vi "Clean Up Actor.vi"(8 "error in (no error)":errorcluster, 11 "User Interface in":refnum<class "User Interface.lvclass">) -> (0 "error out":errorcluster, 3 "User Interface out":refnum<class "User Interface.lvclass">)   [LabVIEW 2016, in "CLD Exam - ATM.lvlib" / "User Interface.lvclass"]
uses:
  User Interface.lvclass
  D:/Repos/Stream/software/Mediator/Classes/Mediated Actor/Mediated Actor.lvclass
  Mediator/Classes/Message Broker Interface/Message Broker Interface.lvclass
  Mediator/Classes/Mediated Synchronous Actor/Mediated Synchronous Actor.lvclass
  Mediator/Classes/Mediated Actor/Mediated Actor.lvclass
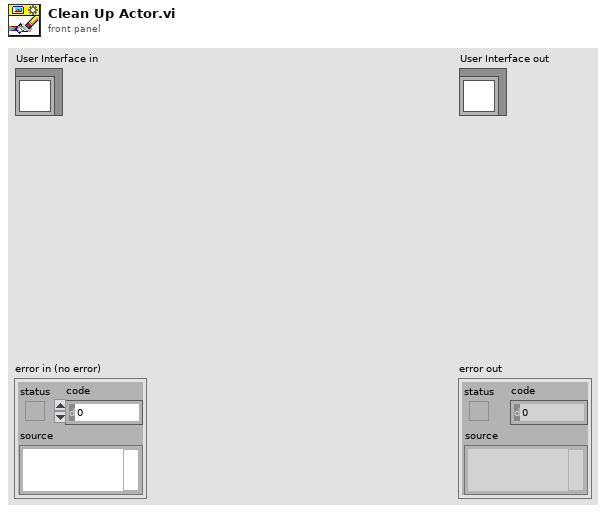
[diagram p1: front panel]
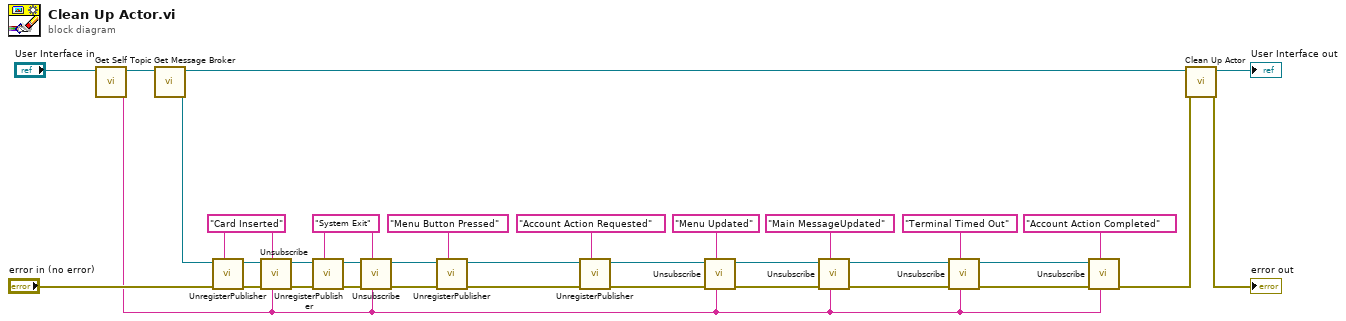
[diagram p0: block diagram]
diagram:
  w25 = "System Exit" ("Topic Name")
  w30 = "Card Inserted" ("Topic Name")
  n1 = call "Get Self Topic.vi"("Mediated Actor in"="User Interface in") -> ("Topic.Self"=w1:string, "Mediated Actor out"=w29:refnum<class "User Interface.lvclass">)  [unwired: 9 in]
  n2 = call "Get Message Broker.vi"("Mediated Actor in"=w29) -> ("Message Broker"=w33:refnum<class "Message Broker Interface.lvclass">, "Mediated Actor out"=w27:refnum<class "User Interface.lvclass">)  [unwired: 9 in]
  n3 = call-dynamic "UnregisterPublisher.vi"("Topic Name"=w30, "error in (no error)"="error in (no error)", "Message Broker Interface in"=w33) -> ("error out"=w31:errorcluster, "Message Broker Interface out"=w32:refnum<class "Message Broker Interface.lvclass">)  [unwired: 7 in]
  n4 = call-dynamic "Unsubscribe.vi"("Subscriber Name"=w1, "Topic Name"=w30, "error in (no error)"=w31, "Message Broker Interface in"=w32) -> ("error out"=w22:errorcluster, "Message Broker Interface out"=w21:refnum<class "Message Broker Interface.lvclass">)  [unwired: 6 in]
  n5 = call-dynamic "UnregisterPublisher.vi"("Topic Name"=w25, "error in (no error)"=w22, "Message Broker Interface in"=w21) -> ("error out"=w24:errorcluster, "Message Broker Interface out"=w23:refnum<class "Message Broker Interface.lvclass">)  [unwired: 7 in]
  n6 = call-dynamic "Unsubscribe.vi"("Subscriber Name"=w1, "Topic Name"=w25, "error in (no error)"=w24, "Message Broker Interface in"=w23) -> ("error out"=w19:errorcluster, "Message Broker Interface out"=w20:refnum<class "Message Broker Interface.lvclass">)  [unwired: 6 in]
  n7 = call-dynamic "UnregisterPublisher.vi"("Topic Name"="Menu Button Pressed", "error in (no error)"=w19, "Message Broker Interface in"=w20) -> ("error out"=w6:errorcluster, "Message Broker Interface out"=w7:refnum<class "Message Broker Interface.lvclass">)  [unwired: 7 in]
  n8 = call-dynamic "UnregisterPublisher.vi"("Topic Name"="Account Action Requested", "error in (no error)"=w6, "Message Broker Interface in"=w7) -> ("error out"=w8:errorcluster, "Message Broker Interface out"=w9:refnum<class "Message Broker Interface.lvclass">)  [unwired: 7 in]
  n9 = call-dynamic "Unsubscribe.vi"("Subscriber Name"=w1, "Topic Name"="Menu Updated", "error in (no error)"=w8, "Message Broker Interface in"=w9) -> ("error out"=w11:errorcluster, "Message Broker Interface out"=w12:refnum<class "Message Broker Interface.lvclass">)  [unwired: 6 in]
  n10 = call-dynamic "Unsubscribe.vi"("Subscriber Name"=w1, "Topic Name"="Main MessageUpdated", "error in (no error)"=w11, "Message Broker Interface in"=w12) -> ("error out"=w13:errorcluster, "Message Broker Interface out"=w14:refnum<class "Message Broker Interface.lvclass">)  [unwired: 6 in]
  n11 = call-dynamic "Unsubscribe.vi"("Subscriber Name"=w1, "Topic Name"="Terminal Timed Out", "error in (no error)"=w13, "Message Broker Interface in"=w14) -> ("error out"=w3:errorcluster, "Message Broker Interface out"=w4:refnum<class "Message Broker Interface.lvclass">)  [unwired: 6 in]
  n12 = call-dynamic "Unsubscribe.vi"("Subscriber Name"=w1, "Topic Name"="Account Action Completed", "error in (no error)"=w3, "Message Broker Interface in"=w4) -> ("error out"=w2:errorcluster)  [unwired: 6 in, 1 out]
  n13 = call-parent "Clean Up Actor.vi"("error in (no error)"=w2, "Mediated Actor in"=w27) -> ("error out"=→"error out":errorcluster, "Mediated Actor out"=→"User Interface out":refnum<class "User Interface.lvclass">)  [unwired: 8 in]
